vi "CameraSetScaledAttr.vi"(8 "error in":errorcluster, 9 "Scaled":dbl, 10 "Attr String":string, 11 "IMAQdx Session in":T1) -> (0 "error out":errorcluster, 3 "IMAQdx Session":T1)   [LabVIEW 2025]
doc: "This VI updates an attribute where input unit is percentage and camera parameter may be in another unit.\n\nThis software is licensed. Open the labview\\readme\\WPI Robotics Library Open Source License.txt file for more information."
uses:
  <vilib>/userDefined/High Color/IMAQdx.ctl
  <resource>/objmgr/imaqdx.rc
panel:
  out "element":dbl
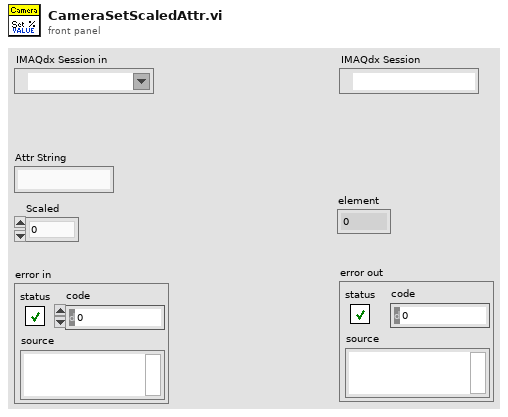
[diagram p1: front panel]
types:
  T1 = typedef "IMAQdx.ctl" = refnum<k21>
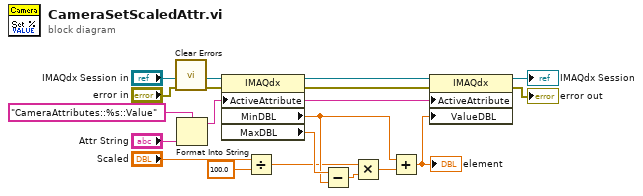
[diagram p0: block diagram]
diagram:
  n1 = call <vilib>:"Clear Errors.vi"("error in (no error)"="error in") -> ("error out"=w10:errorcluster)  [unwired: 5 in, 1 out]
  n2 = Format Into String(format string="CameraAttributes::%s::Value" ("Attr Format"), "Attr String") -> (resulting string=w15:string)  [unwired: 2 in, 1 out]
  n3 = property class="IMAQdx"(reference="IMAQdx Session in", error in=w10, "ActiveAttribute"=w15) -> (reference out=w13:T1, error out=w11:errorcluster, "MinDBL"=w6:dbl, "MaxDBL"=w8:dbl)
  n4 = Divide(x="Scaled", y=100.0) -> (x/y=w2:dbl)
  n5 = Subtract(x=w8, y=w6) -> (x-y=w7:dbl)
  n6 = Multiply(x=w2, y=w7) -> (x*y=w5:dbl)
  n7 = Add(x=w6, y=w5) -> (x+y=w4:dbl)
  "element" <- w4
  n8 = property class="IMAQdx"(reference=w13, error in=w11, "ActiveAttribute"=w15, "ValueDBL"=w4) -> (reference out=→"IMAQdx Session":T1, error out=→"error out":errorcluster)
